vi "Set Node Label.vi"(10 "Node Label":string, 11 "Node in":variant) -> (3 "Node out":variant)   [LabVIEW 2021, in "GraphLib.lvlib" / "Abstract Graph.lvclass"]
uses:
  Abstract Graph.lvclass
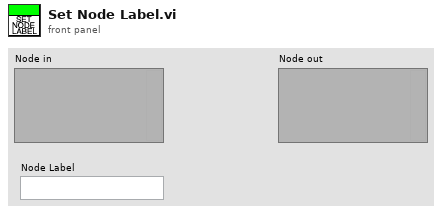
[diagram p1: front panel]
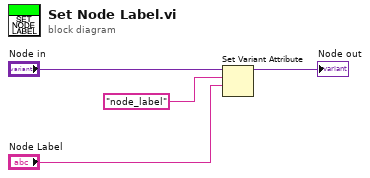
[diagram p0: block diagram]
diagram:
  n1 = Set Variant Attribute(Variant="Node in", name="node_label", value="Node Label") -> (Variant out=→"Node out":variant)  [unwired: 1 in, 2 out]
